vi "convert_string_to_int32.vi"(3 "default (0)":i32, 4 "String in":string) -> (1 "int32 value out":i32)   [LabVIEW 2022 SP3, in "hmp4000_rsidr_core.lvlib"]
uses:
  hmp4000_rsidr_core.lvlib
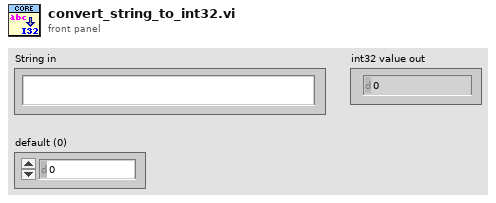
[diagram p1: front panel]
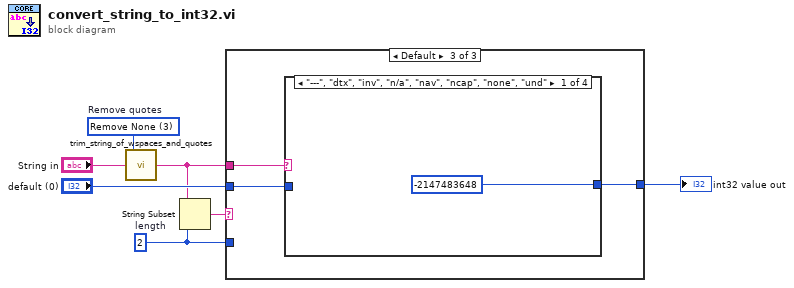
[diagram p0: block diagram]
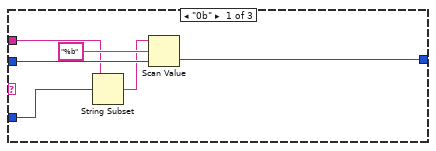
[diagram p2: hidden frame]
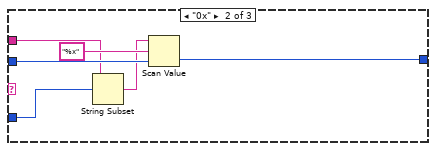
[diagram p3: hidden frame]
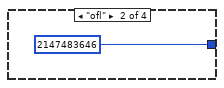
[diagram p4: hidden frame]
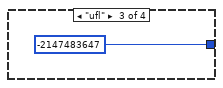
[diagram p5: hidden frame]
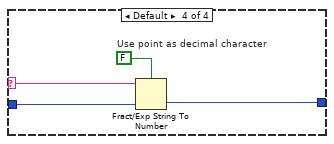
[diagram p6: hidden frame]
diagram:
  w1 = u16 3 items=["Remove All Quotes", "Remove Single Quotes", "Remove Double Quotes", "Remove None"]  # Remove quotes
  w4 = 2  # length
  n1 = call "trim_string_of_wspaces_and_quotes.vi"("String in"="String in", "Remove quotes (Remove All)"=w1) -> ("String out"=w2:string)  [unwired: 3 in]
  n2 = String Subset(string=w2, length (rest)=w4) -> (substring=w5:string)  [unwired: 1 in]
  n3 = case shown="Default" w5 {
    tunnel: [w13 w19 w20] -> w7
    tunnel: w2 -> [w9 w15 w22]
    tunnel: "default (0)" -> [w12 w18 w21]
    tunnel: w4 -> [w10 w16 _]
    frame "0b" {
      n4 = String Subset(string=w9, offset (0)=w10) -> (substring=w8:string)  [unwired: 1 in]
      n5 = Scan Value(string=w8, format string="%b", default (0 dbl)=w12) -> (value=w13:i32)  [unwired: 1 out]
    }
    frame "0x" {
      n6 = String Subset(string=w15, offset (0)=w16) -> (substring=w14:string)  [unwired: 1 in]
      n7 = Scan Value(string=w14, format string="%x", default (0 dbl)=w18) -> (value=w19:i32)  [unwired: 1 out]
    }
    frame Default {
      n8 = case shown="\"---\", \"dtx\", \"inv\", \"n/a\", \"nav\", \"ncap\", \"none\", \"und\"" w22 {
        selector: w22 -> [_ _ _ w26]
        tunnel: w21 -> [_ _ _ w29]
        tunnel: [-2147483648 2147483646 -2147483647 w28] -> w20
        frame "---", "dtx", "inv", "n/a", "nav", "ncap", "none", "und" {
        }
        frame "ofl" {
        }
        frame "ufl" {
        }
        frame Default {
          w27 = FALSE  # Use point as decimal character
          n9 = Fract/Exp String To Number(use system decimal point (T)=w27, string=w26, default (0 dbl)=w29) -> (number=w28:i32)  [unwired: 1 in, 1 out]
        }
      }
    }
  }
  "int32 value out" <- w7
